vi "AdcConversion.vi"(8 "error in (no error)":errorcluster, 11 "Multi Channel ADC in":refnum<class "Multi Channel ADC.lvclass">) -> (0 "error out":errorcluster, 2 "ADC U8 Array":u8[](array[numeric]), 3 "Multi Channel ADC out":refnum<class "Multi Channel ADC.lvclass">)   [LabVIEW 2023, in "Multi Channel ADC.lvclass"]
uses:
  Multi Channel ADC.lvclass
  C:/Users/santharu.subramanian/Documents/ADC_SDLC/ADC_SDLC/Adc/Classes/Conversion/Conversion.lvclass
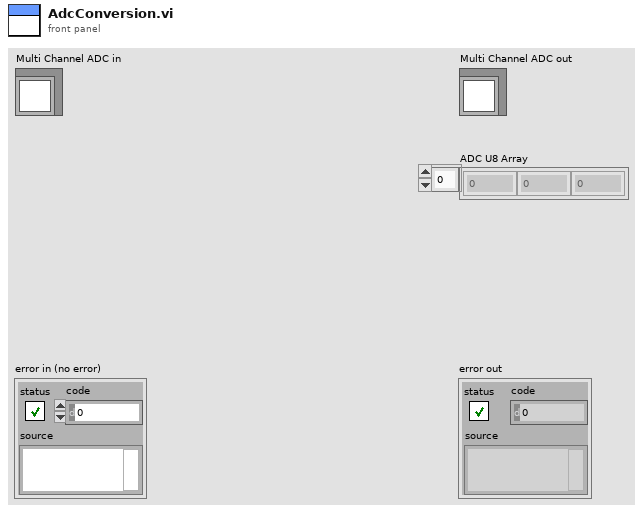
[diagram p1: front panel]
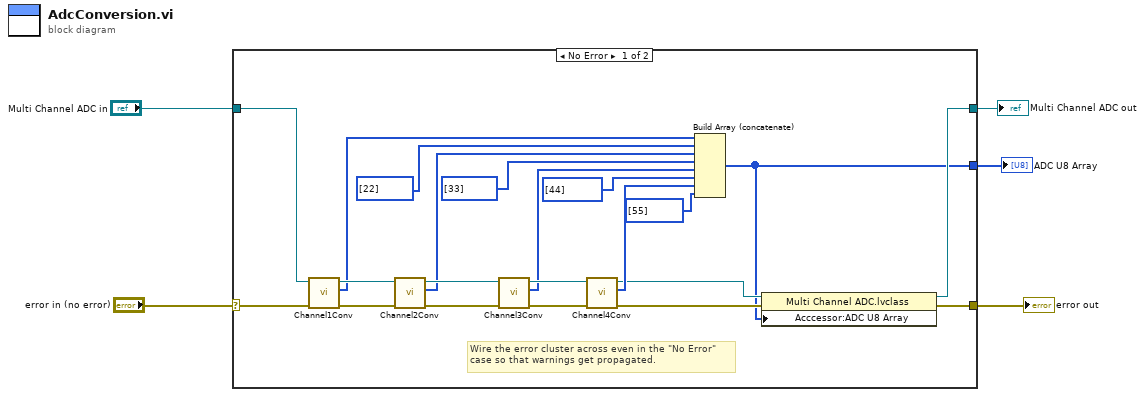
[diagram p0: block diagram]
diagram:
  n1 = case shown="No Error" "error in (no error)" {
    selector: "error in (no error)" -> [w26 w28]
    tunnel: [w9 w28] -> w4
    tunnel: [w7 w27] -> w2
    tunnel: "Multi Channel ADC in" -> [w18 w27]
    tunnel: [w6 _] -> w1
    frame No Error {
      # "Wire the error cluster across even in the \"No Error\"\ncase so that warnings get propagated."
      n2 = call "Channel1Conv.vi"("error in (no error)"=w26, "Multi Channel ADC in"=w18) -> ("error out"=w24:errorcluster, "Channel 1 U8 Array"=w17:u8[], "Multi Channel ADC out"=w25:refnum<class "Multi Channel ADC.lvclass">)  [unwired: 7 in]
      n3 = call "Channel2Conv.vi"("error in (no error)"=w24, "Multi Channel ADC in"=w25) -> ("error out"=w22:errorcluster, "Channel 2 U8 Array"=w16:u8[], "Multi Channel ADC out"=w23:refnum<class "Multi Channel ADC.lvclass">)  [unwired: 7 in]
      n4 = call "Channel3Conv.vi"("error in (no error)"=w22, "Multi Channel ADC in"=w23) -> ("error out"=w20:errorcluster, "Channel 3 U8 Array"=w15:u8[], "Multi Channel ADC out"=w21:refnum<class "Multi Channel ADC.lvclass">)  [unwired: 7 in]
      n5 = call "Channel4Conv.vi"("error in (no error)"=w20, "Multi Channel ADC in"=w21) -> ("error out"=w19:errorcluster, "Channel 4 U8 Array"=w14:u8[], "Multi Channel ADC out"=w8:refnum<class "Multi Channel ADC.lvclass">)  [unwired: 7 in]
      n6 = Build Array (concatenate)(w17, u8[] [22] ("array"), w16, u8[] [33] ("array"), w15, u8[] [44] ("array"), w14, u8[] [55] ("array")) -> (w6:u8[])
      n7 = property class="Multi Channel ADC.lvclass"(reference=w8, error in=w19, "Acccessor:ADC U8 Array"=w6) -> (reference out=w7:refnum<class "Multi Channel ADC.lvclass">, error out=w9:errorcluster)
    }
    frame Error {
    }
  }
  "error out" <- w4
  "Multi Channel ADC out" <- w2
  "ADC U8 Array" <- w1
